vi "wal checkpoint v2.vi"(0 "db":dbl, 1 "pnCkpt":i32, 5 "zDb":string, 7 "eMode":i32, 9 "pnLog":i32, 11 "error in (no error)":errorcluster) -> (3 "pnCkpt out":i32, 4 "db out":dbl, 6 "function return":i32, 10 "pnLog out":i32, 15 "error out":errorcluster)   [LabVIEW 2020, in "sqlite3.lvlib"]
uses:
  sqlite3.lvlib
  errstr.vi
  bin/sqlite3_64.dll
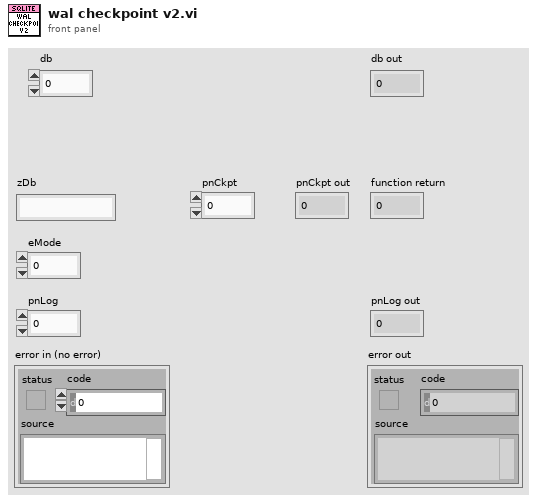
[diagram p1: front panel]
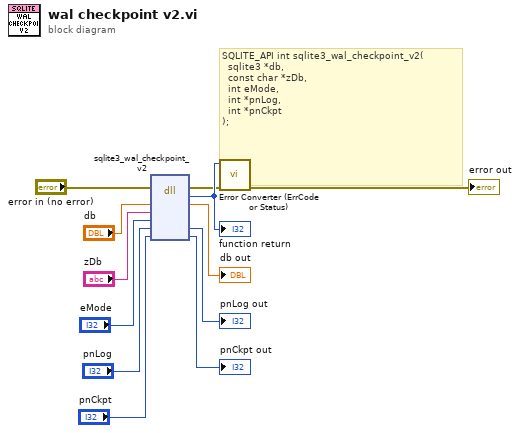
[diagram p0: block diagram]
diagram:
  # "SQLITE_API int sqlite3_wal_checkpoint_v2(\n  sqlite3 *db,                    \n  const char *zDb,                \n  int eMode,                      \n  int *pnLog,                     \n  int *pnCkpt                     \n);"
  n1 = dll-call lib="D:/Project/Labview-Projects/database-configuration/externals/sqlite3/Source/bin/sqlite3_*.*" fn="sqlite3_wal_checkpoint_v2"(error in="error in (no error)", "db"="db", "zDb"="zDb", "eMode"="eMode", "pnLog"="pnLog", "pnCkpt"="pnCkpt") -> (error out=w2:errorcluster, w12:i32, "db"=→"db out":dbl, "pnLog"=→"pnLog out":i32, "pnCkpt"=→"pnCkpt out":i32)  [unwired: 4 in, 1 out]
  "function return" <- w12
  n2 = call "Error Converter (ErrCode or Status).vi"("error in (no error)"=w2, "error code"=w12) -> ("error out"=→"error out":errorcluster)  [unwired: 9 in]
